vi "EFMC-ZMB.vi"() -> (1 "GNSS2卫星禁用控制状态":string caption="GNSS2卫星", 2 "GNSS1卫星禁用控制状态":string caption="GNSS1卫星", 3 "飞机安装-识别码":string caption="识别码", 4 "星敏1-识别码":string caption="识别码", 6 "组合模式控制设置状态":string caption="组合模式", 8 "星敏2-识别码":string caption="识别码", 10 "GNSS3卫星禁用控制状态":string caption="GNSS3卫星")   [LabVIEW 2012]
uses:
  <vilib>/GPower/VIRegister/Library/Convert/ToStr.vi
  <vilib>/GPower/VIRegister/Library/SubVIs/FindRegisterData.vi
  <vilib>/GPower/VIRegister/Library/SubVIs/ReadSub.vi
  <vilib>/GPower/VIRegister/Library/QManager/GetRegisterData.vi
  <vilib>/GPower/Error/Library/SetError.vi
  <vilib>/GPower/Error/Library/FilterCodes.vi
  <vilib>/GPower/Error/Library/Filter/FilterMulti.vi
  <vilib>/GPower/VIRegister/Library/QManager/QManagerAction.vi
  <vilib>/GPower/Error/Library/ErrorType.vi
  <vilib>/GPower/Error/Library/SplitAppended.vi
  <vilib>/GPower/Error/Library/SubVIs/ExplanationToError.vi
  <vilib>/GPower/VIRegister/Library/QManager/GetQName.vi
  <vilib>/GPower/VIRegister/Library/QManager/StartQManager.vi
  <vilib>/Utility/error.llb/Trim Whitespace.vi
  <vilib>/dlg_ctls.llb/Space Constant.vi
  <vilib>/Utility/error.llb/Error Code Database.vi
  <vilib>/GPower/Error/Library/SubVIs/SetStatus.vi
  <vilib>/GPower/Error/Library/AppendErrors.vi
  <vilib>/GPower/Error/Library/Append/AppendSingle.vi
  <vilib>/GPower/VIRegister/VIRegister.lvlib
panel:
  out "星敏2-偏航角修正值":i16 caption="偏航角修正值"
  out "星敏2-滚转角修正值":i16 caption="滚转角修正值"
  out "星敏2-俯仰角修正值":i16 caption="俯仰角修正值"
  out "星敏1-偏航角修正值":i16 caption="偏航角修正值"
  out "星敏1-滚转角修正值":i16 caption="滚转角修正值"
  out "星敏1-俯仰角修正值":i16 caption="俯仰角修正值"
  out "飞机安装-偏航角修正值":i16 caption="偏航角修正值"
  out "飞机安装-滚转角修正值":i16 caption="滚转角修正值"
  out "飞机安装-俯仰角修正值":i16 caption="俯仰角修正值"
  # "修正值"
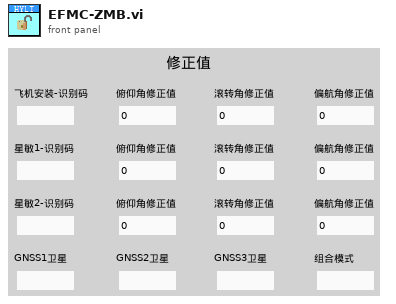
[diagram p1: front panel]
types:
  T1 = cluster{"俯仰角修正值":i16, "滚转角修正值":i16, "偏航角修正值":i16}
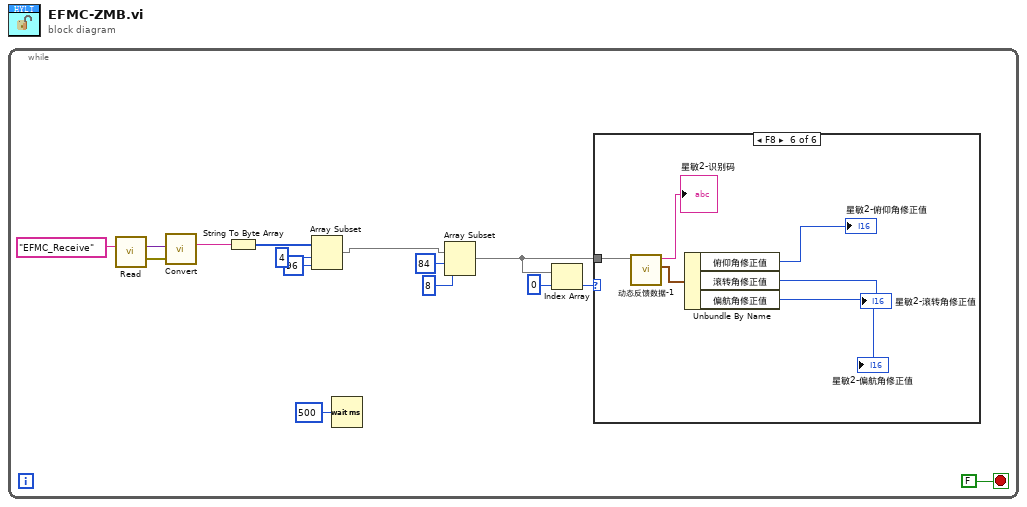
[diagram p0: block diagram]
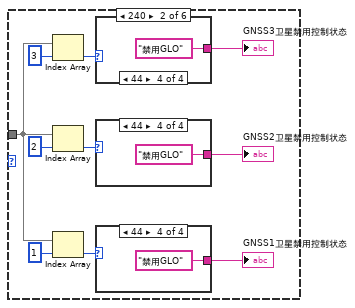
[diagram p3: hidden frame]
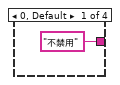
[diagram p4: hidden frame]
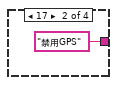
[diagram p5: hidden frame]
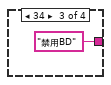
[diagram p6: hidden frame]
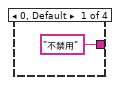
[diagram p7: hidden frame]
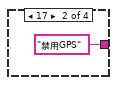
[diagram p8: hidden frame]
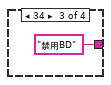
[diagram p9: hidden frame]
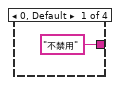
[diagram p10: hidden frame]
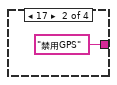
[diagram p11: hidden frame]
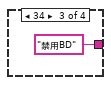
[diagram p12: hidden frame]
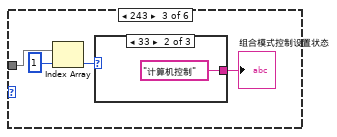
[diagram p13: hidden frame]
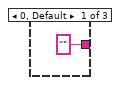
[diagram p14: hidden frame]
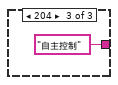
[diagram p15: hidden frame]
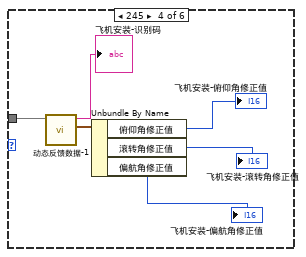
[diagram p16: hidden frame]
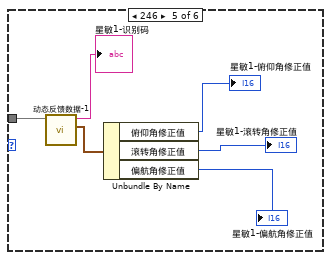
[diagram p17: hidden frame]
diagram:
  n1 = while {
    stop <- FALSE stop-if-true
    n2 = call <vilib>:"Read.vi"("Register name"="EFMC_Receive") -> ("Register value"=w4:variant, "Error out"=w5:errorcluster)  [unwired: 11 in, 2 out]
    n3 = call-poly <vilib>:"Convert.vi"("Register value in"=w4, "Error in"=w5) -> ("Register value out"=w7:string)  [unwired: 12 in, 1 out]
    n4 = String To Byte Array(string=w7) -> (unsigned byte array=w9:u8[])
    n5 = Array Subset(array=w9, index=4 ("索引"), length=96 ("长度")) -> (w3:u8[])
    n6 = Wait (ms)(milliseconds to wait=u32 500 ("等待时间（毫秒）")) -> ()  [unwired: 1 out]
    n7 = Array Subset(array=w3, index=84 ("索引"), length=8 ("长度")) -> (w11:u8[])
    n8 = Index Array(array=w11, index=0 ("索引")) -> (element=w15:u8)
    n9 = case shown="F8" w15 {
      tunnel: w11 -> [_ w16 w40 w50 w55 w61]
      frame 0, Default {
      }
      frame 240 {
        n10 = Index Array(array=w16, index=3 ("索引")) -> (element=w18:u8)
        n11 = Index Array(array=w16, index=2 ("索引")) -> (element=w21:u8)
        n12 = Index Array(array=w16, index=1 ("索引")) -> (element=w24:u8)
        n13 = case shown="44" w18 {
          tunnel: ["不禁用" ("字符串") "禁用GPS" ("字符串") "禁用BD" ("字符串") "禁用GLO" ("字符串")] -> w19
          frame 0, Default {
          }
          frame 17 {
          }
          frame 34 {
          }
          frame 68 {
          }
        }
        "GNSS3卫星禁用控制状态" <- w19
        n14 = case shown="44" w21 {
          tunnel: ["不禁用" ("字符串") "禁用GPS" ("字符串") "禁用BD" ("字符串") "禁用GLO" ("字符串")] -> w20
          frame 0, Default {
          }
          frame 17 {
          }
          frame 34 {
          }
          frame 68 {
          }
        }
        "GNSS2卫星禁用控制状态" <- w20
        n15 = case shown="44" w24 {
          tunnel: ["不禁用" ("字符串") "禁用GPS" ("字符串") "禁用BD" ("字符串") "禁用GLO" ("字符串")] -> w25
          frame 0, Default {
          }
          frame 17 {
          }
          frame 34 {
          }
          frame 68 {
          }
        }
        "GNSS1卫星禁用控制状态" <- w25
      }
      frame 243 {
        n16 = Index Array(array=w40, index=1 ("索引")) -> (element=w39:u8)
        n17 = case shown="33" w39 {
          tunnel: ["" ("字符串") "计算机控制" ("字符串") "自主控制" ("字符串")] -> w41
          frame 0, Default {
          }
          frame 51 {
          }
          frame 204 {
          }
        }
        "组合模式控制设置状态" <- w41
      }
      frame 245 {
        n18 = call "动态反馈数据-1.vi"("数组"=w50) -> ("修正值"=w48:T1, "飞机安装-识别码"=→"飞机安装-识别码":string)  [unwired: 9 in]
        n19 = Unbundle By Name(w48) -> ("俯仰角修正值"=→"飞机安装-俯仰角修正值":i16, "滚转角修正值"=→"飞机安装-滚转角修正值":i16, "偏航角修正值"=→"飞机安装-偏航角修正值":i16)
      }
      frame 246 {
        n20 = call "动态反馈数据-1.vi"("数组"=w55) -> ("修正值"=w54:T1, "飞机安装-识别码"=→"星敏1-识别码":string)  [unwired: 9 in]
        n21 = Unbundle By Name(w54) -> ("俯仰角修正值"=→"星敏1-俯仰角修正值":i16, "滚转角修正值"=→"星敏1-滚转角修正值":i16, "偏航角修正值"=→"星敏1-偏航角修正值":i16)
      }
      frame 248 {
        n22 = call "动态反馈数据-1.vi"("数组"=w61) -> ("修正值"=w60:T1, "飞机安装-识别码"=→"星敏2-识别码":string)  [unwired: 9 in]
        n23 = Unbundle By Name(w60) -> ("俯仰角修正值"=→"星敏2-俯仰角修正值":i16, "滚转角修正值"=→"星敏2-滚转角修正值":i16, "偏航角修正值"=→"星敏2-偏航角修正值":i16)
      }
    }
  }
